vi "Keithley6221_PulseDeltaRead.vi"(7 "error in (no error)":errorcluster, 10 "GPIB ADR":u16) -> (0 "error out":errorcluster, 2 "Reading":dbl, 3 "Pulse Delta Current High":dbl)   [LabVIEW 2012]
panel:
  out "VISA Refnum out":refnum<visa-resource-name>
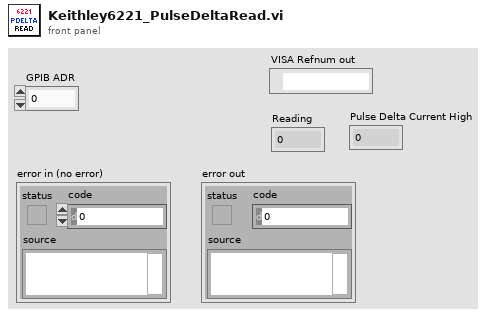
[diagram p1: front panel]
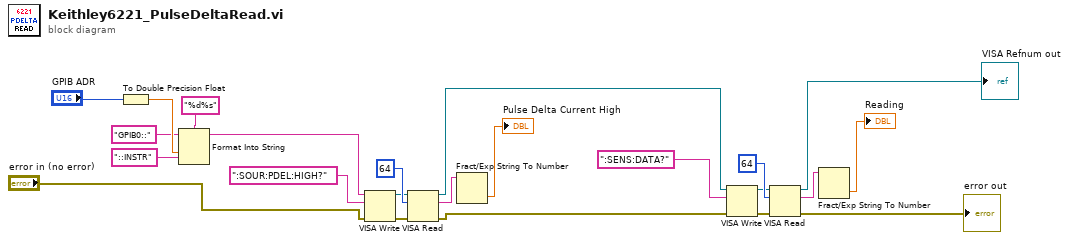
[diagram p0: block diagram]
diagram:
  n1 = To Double Precision Float(number="GPIB ADR") -> (double precision float=w14:dbl)
  n2 = Format Into String(format string="%d%s" ("Removes all labels from the string"), initial string="GPIB0::", w14, "::INSTR") -> (resulting string=w2:string)  [unwired: 1 in, 1 out]
  n3 = VISA Write(VISA resource name=w2, write buffer=":SOUR:PDEL:HIGH?", error in (no error)="error in (no error)") -> (VISA resource name out=w6:refnum<visa-resource-name>, error out=w8:errorcluster)  [unwired: 1 out]
  n4 = VISA Read(VISA resource name=w6, byte count=u32 64, error in (no error)=w8) -> (VISA resource name out=w4:refnum<visa-resource-name>, read buffer=w9:string, error out=w3:errorcluster)  [unwired: 1 out]
  n5 = Fract/Exp String To Number(string=w9) -> (number=→"Pulse Delta Current High":dbl)  [unwired: 3 in, 1 out]
  n6 = VISA Write(VISA resource name=w4, write buffer=":SENS:DATA?", error in (no error)=w3) -> (VISA resource name out=w17:refnum<visa-resource-name>, error out=w19:errorcluster)  [unwired: 1 out]
  n7 = VISA Read(VISA resource name=w17, byte count=u32 64, error in (no error)=w19) -> (VISA resource name out=→"VISA Refnum out":refnum<visa-resource-name>, read buffer=w22:string, error out=→"error out":errorcluster)  [unwired: 1 out]
  n8 = Fract/Exp String To Number(string=w22) -> (number=→"Reading":dbl)  [unwired: 3 in, 1 out]
